vi "Audio Test.Stepped Sine Sweep Analysis.vi"(7 "SigConfig":refnum<class "SV Discrete Sweep.lvclass">=refnum, 8 "error in":errorcluster, 9 "StepCnt":i32, 10 "Response Wvfrm":waveform(dbl), 11 "Stimulus Wvfrm":waveform(dbl)) -> (0 "error out":errorcluster, 2 "THD":cluster{"frequency":dbl[], "THD":dbl[]}(graph), 3 "Magnitude":cluster{"frequency":dbl[], "magnitude":dbl[]}(graph))   [LabVIEW 2018]
uses:
  <vilib>/addons/Sound and Vibration/svt_Level/SVL AC & DC Level (Time) (1 Ch).vi
  <vilib>/addons/_NISVFA/_Shared subVIs/Data Objects/Waveforms (DBL)/Waveforms (N Ch).lvclass
  Common/Utils/Errors/Error.Error Code List.ctl
  <vilib>/addons/Sound and Vibration/svt_Single Tone Measurements/SVT Gain and Phase (Time).vi
  <vilib>/addons/Sound and Vibration/svt_Distortion/SVT THD and Harmonic Components (Frequency) (1 Ch).vi
  <vilib>/addons/_NISVFA/_Shared subVIs/Common/SV Append Data (N Ch) (DBL).vi
  <vilib>/addons/_NISVFA/_Shared subVIs/Data Objects/Waveforms (DBL)/SV Read Next Measurement Data.vi
  <vilib>/addons/_NISVFA/_Generation/Signal Generation/SV Discrete Sweep/SV Discrete Sweep.lvclass
panel:
  in  "Boolean":bool
  in  "t0":timestamp=timestamp(3624589532.907914 s since 1904-01-01) format="%<%X\n%x>T"
  out "Waveform Graph 2":waveform(dbl)(graph)
  out "Waveform Graph":waveform(dbl)(graph)
  out "Play dt":dbl
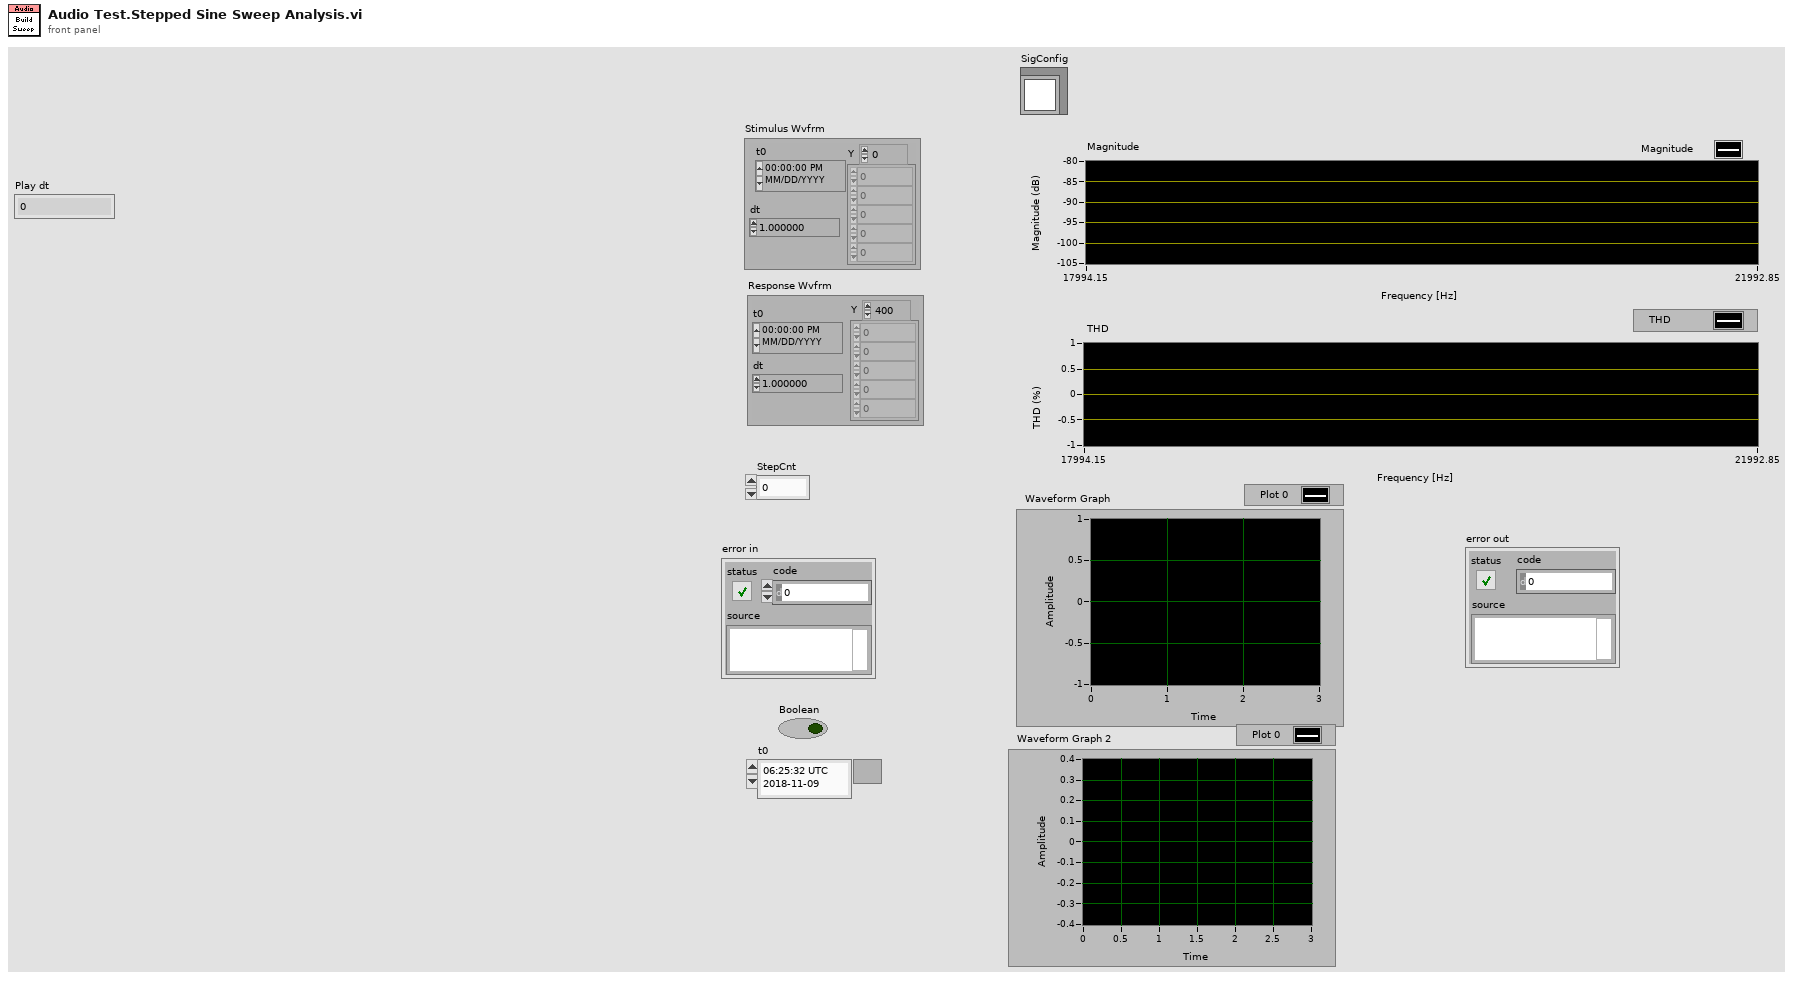
[diagram p1: front panel]
types:
  T1 = cluster{"gain units":enum16{"dB", "linear ratio"}, "phase units":enum16{"deg", "rad"}, "detected tone stimulus amplitude units":enum16{"EU rms", "EU peak", "EU peak-peak"}, "detected tone response amplitude units":enum16{"EU rms", "EU peak", "EU peak-peak"}}
  T2 = cluster{"THD units":enum16{"dB", "linear ratio", "%"}, "harmonic component amplitude units":enum16{"EU rms", "EU peak", "EU peak-peak", "dB ref fund"}, "detected fundamental amplitude units":enum16{"EU rms", "EU peak", "EU peak-peak"}}
  T3 = typedef "svc_Spectrum Info.ctl" = cluster{"channel name":string, "description":string, "x-axis units":T4, "spectral info":cluster{"spectrum type":T5, "linear/dB":enum16{"linear", "dB"}, "window":u16, "window size":i32, "FFT size":i32}, "engineering units":T6, "custom label":string, "dB reference [EU]":dbl, "peak units":enum16{"rms", "peak", "peak-peak"}, "weighting filter":T7, "spectral density?":bool, "unit label":string, "spectrum skewed?":bool, "complimentary spectrum units":T8}
  T4 = typedef "svc_X-Axis Units.ctl" = u16
  T5 = typedef "svc_Spectrum Type.ctl" = enum16{"FFT Spectrum [complex]", "Amplitude [Magnitude]", "Power [Magnitude^2]", "Cross Spectrum [complex]", "Frequency Response [Complex]"}
  T6 = typedef "svc_Engineering Units Text Ring.ctl" = u16
  T7 = typedef "svc_Weighting Filter Text Ring.ctl" = u16
  T8 = typedef "svc_Complimentary Spectrum Units.ctl" = enum16{"none", "radians", "degrees", "cycles", "imaginary"}
  T9 = cluster{"complex spectrum response":cluster{"f0":dbl, "df":dbl, "complex spectrum":cdb[]}, "spectrum info":T3}
  T10 = typedef "Error.Error Code List.ctl" = i32
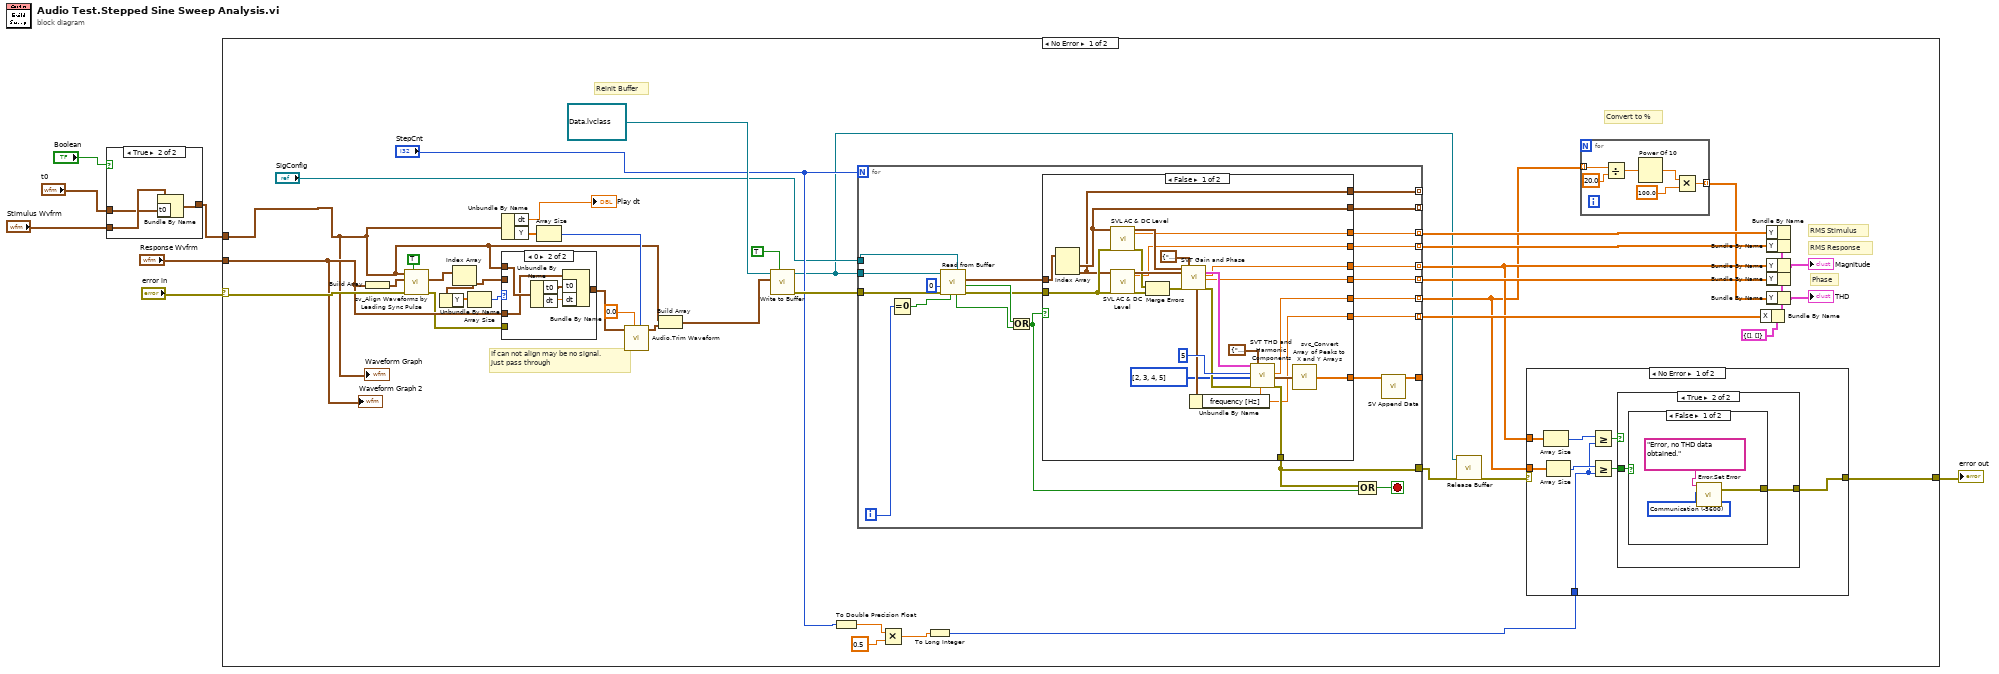
[diagram p0: block diagram]
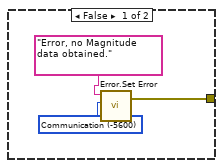
[diagram p4: hidden frame]
diagram:
  n1 = case shown="True" "Boolean" {
    tunnel: "Stimulus Wvfrm" -> [w8 w11]
    tunnel: [w8 w10] -> w3
    tunnel: "t0" -> [_ w9]
    frame False {
    }
    frame True {
      n2 = Bundle By Name(cluster=w11, "t0"=w9) -> (w10:waveform(dbl))
    }
  }
  n3 = case shown="No Error" "error in" {
    selector: "error in" -> [w30 w130]
    tunnel: w3 -> [w18 _]
    tunnel: "Response Wvfrm" -> [w29 _]
    tunnel: [w31 w130] -> w6
    frame No Error {
      # "If can not align may be no signal.\nJust pass through"
      # "Convert to %"
      # "Reinit Buffer"
      # "RMS Response"
      # "RMS Stimulus"
      # "Phase"
      n4 = Build Array(w29) -> (w51:waveform(dbl)[])
      n5 = call "sv_Align Waveforms by Leading Sync Pulse.vi"("reset"=TRUE, "error in (no error)"=w30, "response signals"=w51, "alignment reference signal"=w18) -> ("error out"=w24:errorcluster, "aligned signals"=w28:waveform(dbl)[])  [unwired: 3 in, 3 out]
      n6 = Index Array(array=w28) -> (element=w26:waveform(dbl))  [unwired: 1 in]
      n7 = Unbundle By Name(w26) -> ("Y"=w27:dbl[])
      n8 = Array Size(array=w27) -> (size(s)=w25:i32)
      n9 = case shown="0" w25 {
        tunnel: [w53 w57] -> w50
        tunnel: w26 -> [w53 _]
        tunnel: w29 -> [_ w54]
        tunnel: w18 -> [_ w58]
        tunnel: w24 -> [_ _]
        frame Default {
        }
        frame 0 {
          n10 = Unbundle By Name(w58) -> ("t0"=w56:timestamp, "dt"=w55:dbl)
          n11 = Bundle By Name(cluster=w54, "t0"=w56, "dt"=w55) -> (w57:waveform(dbl))
        }
      }
      n12 = Unbundle By Name(w18) -> ("dt"=→"Play dt":dbl, "Y"=w48:dbl[])
      n13 = Array Size(array=w48) -> (size(s)=w46:i32)
      n14 = call "Audio.Trim Waveform.vi"("Len"=w46, "Max Delay"=0.0, "Data In"=w50) -> ("Data Out"=w47:waveform(dbl))  [unwired: 8 in]
      n15 = Build Array(w18, w47) -> (w17:waveform(dbl)[])
      n16 = call <vilib>:"Write to Buffer.vi"("clear buffer (False)"=TRUE, "waveforms"=w17, "buffer"=refnum<data-value> refnum) -> ("error out"=w52:errorcluster, "buffer out"=w13:refnum<data-value>)  [unwired: 6 in, 1 out]
      n17 = To Double Precision Float(number="StepCnt") -> (double precision float=w21:dbl)
      n18 = for {
        N: "StepCnt" -> [_]
        tunnel: w13 -> [w103]
        tunnel: "SigConfig" -> [w102]
        tunnel: w52 -> [w101]
        tunnel: [w89] -> w15
        tunnel: [w98] -> w39 mode=indexing
        tunnel: [w97] -> w40 mode=indexing
        tunnel: [w96] -> w34 mode=indexing
        tunnel: [w95] -> w41 mode=indexing
        tunnel: [w94] -> w33 mode=indexing
        tunnel: [w86] -> w43 mode=indexing
        tunnel: [w92] -> _
        tunnel: [w91] -> _ mode=indexing
        tunnel: [w90] -> _ mode=indexing
        i -> [w83]
        stop <- w99 stop-if-true
        n19 = Equal To 0?(x=w83) -> (x = 0?=w84:bool)
        n20 = call-poly <vilib>:"Read from Buffer.vi"("test signal configuration"=w102, "reset start (F)"=w84, "error in (no error)"=w101, "timeout (1000 ms)"=0, "buffer"=w103) -> ("error out"=w82:errorcluster, "end of buffer"=w88:bool, "waveforms subset"=w100:waveform(dbl)[], "done"=w87:bool)  [unwired: 2 in, 1 out]
        n21 = Or(x=w88, y=w87) -> (x .or. y?=w85:bool)
        n22 = case shown="False" w85 {
          tunnel: w82 -> [w129 _]
          tunnel: w100 -> [w128 _]
          tunnel: [w114 _] -> w98
          tunnel: [w113 _] -> w97
          tunnel: [w112 _] -> w96
          tunnel: [w111 _] -> w95
          tunnel: [w110 _] -> w94
          tunnel: [w109 _] -> w93
          tunnel: [w108 _] -> w91
          tunnel: [w107 _] -> w90
          tunnel: [w106 _] -> w89
          tunnel: [w105 _] -> w86
          frame False {
            n23 = Index Array(array=w128) -> (element #1=w108:waveform(dbl), element #2=w107:waveform(dbl))  [unwired: 2 in]
            n24 = call-poly <vilib>:"SVL AC & DC Level.vi"("scaled signal [EU]"=w108, "error in (no error)"=w129) -> ("AC signal [EU]"=w122:waveform(dbl), "AC level [EU rms]"=w114:dbl, "error out"=w119:errorcluster)  [unwired: 12 in, 3 out]
            n25 = call-poly <vilib>:"SVL AC & DC Level.vi"("scaled signal [EU]"=w107, "error in (no error)"=w129) -> ("AC signal [EU]"=w121:waveform(dbl), "AC level [EU rms]"=w113:dbl, "error out"=w118:errorcluster)  [unwired: 12 in, 3 out]
            n26 = Merge Errors(w119, w118) -> (w117:errorcluster)
            n27 = call-poly <vilib>:"SVT Gain and Phase.vi"("stimulus signal X [EUx]"=w122, "response signal Y [EUy]"=w121, "error in (no error)"=w117, "desired units"=T1 {"gain units"=enum."dB", "phase units"=enum."deg", "detected tone stimulus amplitude units"=enum."EU rms", "detected tone response amplitude units"=enum."EU rms"}) -> ("detected tone response"=w116:cluster{"frequency [Hz]":dbl, "amplitude":dbl}, "complex spectrum\nresponse Y"=w123:T9, "gain"=w112:dbl, "phase lag"=w111:dbl, "error out"=w120:errorcluster)  [unwired: 8 in, 3 out]
            n28 = Unbundle By Name(w116) -> ("frequency [Hz]"=w105:dbl)
            n29 = call-poly <vilib>:"SVT THD and Harmonic Components.vi"("complex spectrum"=w123, "maximum harmonic"=5, "harmonics to visualize"=i32[] [2, 3, 4, 5], "error in (no error)"=w120, "desired units"=T2 {"THD units"=enum."dB", "harmonic component amplitude units"=enum."dB ref fund", "detected fundamental amplitude units"=enum."EU peak"}, "expected fundamental frequency [Hz]"=w105) -> ("THD"=w110:dbl, "harmonic components"=w124:cluster{"frequency [Hz]":dbl, "amplitude":dbl}[], "error out"=w106:errorcluster)  [unwired: 6 in, 5 out]
            n30 = call <vilib>:"svc_Convert Array of Peaks to X and Y Arrays.vi"("peaks"=w124) -> ("Y"=w109:dbl[])  [unwired: 3 in, 1 out]
          }
          frame True {
          }
        }
        n31 = Compound Arithmetic op=OR(w89, w85) -> (w99:bool)
        n32 = call-poly <vilib>:"SV Append Data.vi"("data in"=w93) -> ("appended data"=w92:dbl[][])  [unwired: 10 in]
      }
      n33 = Multiply(x=w21, y=0.5) -> (x*y=w22:dbl)
      n34 = To Long Integer(number=w22) -> (32bit integer=w19:i32)
      n35 = call <vilib>:"Release Buffer.vi"("error in (no error)"=w15, "buffer"=w13) -> ("error out"=w14:errorcluster)  [unwired: 9 in]
      n36 = case shown="No Error" w14 {
        selector: w14 -> [_ w81]
        tunnel: w34 -> [w72 _]
        tunnel: w33 -> [w71 _]
        tunnel: [w70 w81] -> w31
        tunnel: w19 -> [w67 _]
        frame No Error {
          n37 = Array Size(array=w72) -> (size(s)=w69:i32)
          n38 = Array Size(array=w71) -> (size(s)=w68:i32)
          n39 = Greater Or Equal?(x=w69, y=w67) -> (x >= y?=w66:bool)
          n40 = Greater Or Equal?(x=w68, y=w67) -> (x >= y?=w65:bool)
          n41 = case shown="True" w66 {
            tunnel: [w73 w77] -> w70
            tunnel: w65 -> [_ w76]
            frame False {
              w74 = T10 -5600 items=["No Error"=0, "Abort"=-2, "Misc"=-5000, "Fixture Error"=-5100, "File IO - General"=-5200, "FIle IO - Config Error"=-5201, "Instrument - General"=-5300, "Instrument - Serial Com"=-5301, "Instrument - Camera"=-5302, "Instrument - PS"=-5303, "Instrument - Oscilloscope"=-5304, "Instrument - Function Gen"=-5305, "Instrument - Load"=-5306, "Instrument - Meter"=-5307, "Instrument - Power Control"=-5308, "Instrument - Motion"=-5309, "Instrument - RF"=-5310, "System Exe"=-5400, "Image Processing"=-5500, "Communication"=-5600, "Script - Syntax Error"=-6000, "Script - Invalid Name or Param"=-6100, "Script - Timeout"=-6200, "Invalid Data"=-6300, "FW Update Error"=-6500] ("Std Code")
              n42 = call "Error.Set Error.vi"("Code"=w74, "Desc"="Error, no Magnitude data obtained.") -> ("error out"=w73:errorcluster)  [unwired: 5 in]
            }
            frame True {
              n43 = case shown="False" w76 {
                tunnel: [w78 _] -> w77
                frame False {
                  w79 = T10 -5600 items=["No Error"=0, "Abort"=-2, "Misc"=-5000, "Fixture Error"=-5100, "File IO - General"=-5200, "FIle IO - Config Error"=-5201, "Instrument - General"=-5300, "Instrument - Serial Com"=-5301, "Instrument - Camera"=-5302, "Instrument - PS"=-5303, "Instrument - Oscilloscope"=-5304, "Instrument - Function Gen"=-5305, "Instrument - Load"=-5306, "Instrument - Meter"=-5307, "Instrument - Power Control"=-5308, "Instrument - Motion"=-5309, "Instrument - RF"=-5310, "System Exe"=-5400, "Image Processing"=-5500, "Communication"=-5600, "Script - Syntax Error"=-6000, "Script - Invalid Name or Param"=-6100, "Script - Timeout"=-6200, "Invalid Data"=-6300, "FW Update Error"=-6500] ("Std Code")
                  n44 = call "Error.Set Error.vi"("Code"=w79, "Desc"="Error, no THD data obtained.") -> ("error out"=w78:errorcluster)  [unwired: 5 in]
                }
                frame True {
                }
              }
            }
          }
        }
        frame Error {
        }
      }
      n45 = for {
        tunnel: w33 -> [w64] mode=indexing
        tunnel: [w59] -> w32 mode=indexing
        n46 = Divide(x=w64, y=20.0) -> (x/y=w62:dbl)
        n47 = Power Of 10(x=w62) -> (10^x=w61:dbl)
        n48 = Multiply(x=w61, y=100.0) -> (x*y=w59:dbl)
      }
      n49 = Bundle By Name(cluster=cluster{"X":dbl[], "Y":dbl[]} {"X"=[], "Y"=[]} ("THD vs Amplitude"), "X"=w43) -> (w44:cluster{"X":dbl[], "Y":dbl[]})
      n50 = Bundle By Name(cluster=w44, "Y"=w39) -> ()  [unwired: 1 out]
      n51 = Bundle By Name(cluster=w44, "Y"=w40) -> ()  [unwired: 1 out]
      n52 = Bundle By Name(cluster=w44, "Y"=w34) -> (→"Magnitude":cluster{"X":dbl[], "Y":dbl[]})
      n53 = Bundle By Name(cluster=w44, "Y"=w41) -> ()  [unwired: 1 out]
      n54 = Bundle By Name(cluster=w44, "Y"=w32) -> (→"THD":cluster{"X":dbl[], "Y":dbl[]})
      "Waveform Graph" <- w18
      "Waveform Graph 2" <- w29
    }
    frame Error {
    }
  }
  "error out" <- w6
